vi "ReadFirmwareVersion.vi"(8 "error in (no error)":errorcluster, 11 "GrovePi in":refnum<class "GrovePi.lvclass">) -> (0 "error out":errorcluster, 2 "Firmware Version":string, 3 "GrovePi out":refnum<class "GrovePi.lvclass">)   [LabVIEW 2014, in "GrovePi.lvclass"]
doc: "Returns the Firmware Version of the GrovePi"
uses:
  GrovePi.lvclass
  Command.ctl
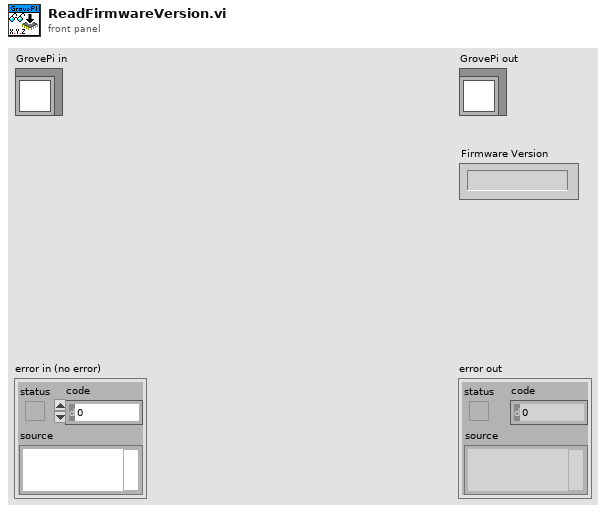
[diagram p1: front panel]
types:
  T1 = typedef "GrovePi.lvclass/Command.ctl" = u8
  T2 = cluster{"Message[0]":u8, "Message[1]":u8, "Message[2]":u8, "Message[3]":u8}
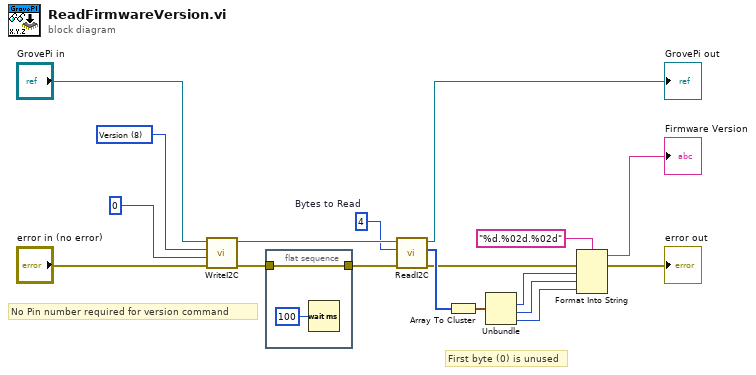
[diagram p0: block diagram]
diagram:
  w11 = u8 4  # Bytes to Read
  w16 = T1 8 items=["Digital Read"=1, "Digital Write"=2, "Analog Read"=3, "Analog Write"=4, "Pin Mode"=5, "Ultrasonic Read"=7, "Version"=8, "Dust Sensor Read"=10, "Encoder Read"=11, "Flow Read"=12, "Flow Disabled"=13, "Dust Sensor Enable"=14, "Dust Sensor Disable"=15, "Encoder Enable"=16, "Encoder Disable"=17, "Flow Enable"=18, "Accelerometer Read"=20, "RTC Read"=30, "DHT Read"=40] ("Command")
  # "First byte (0) is unused"
  # "No Pin number required for version command"
  n1 = call "WriteI2C.vi"("error in (no error)"="error in (no error)", "Pin"=u8 0, "Command"=w16, "GrovePi in"="GrovePi in") -> ("error out"=w14:errorcluster, "GrovePi out"=w12:refnum<class "GrovePi.lvclass">)  [unwired: 5 in, 1 out]
  n2 = flat-sequence {
    tunnel: w14 -> [w19]
    tunnel: [w19] -> w13
    frame #0 {
      n3 = Wait (ms)(milliseconds to wait=u32 100) -> ()  [unwired: 1 out]
    }
  }
  n4 = call "ReadI2C.vi"("error in (no error)"=w13, "Bytes to Read"=w11, "GrovePi in"=w12) -> ("error out"=w7:errorcluster, "Message"=w9:u8[], "GrovePi out"=→"GrovePi out":refnum<class "GrovePi.lvclass">)  [unwired: 6 in]
  n5 = Array To Cluster(array=w9) -> (cluster=w8:T2)
  n6 = Unbundle(w8) -> ("Message[1]"=w3:u8, "Message[2]"=w2:u8, "Message[3]"=w1:u8)  [unwired: 1 out]
  n7 = Format Into String(format string="%d.%02d.%02d", error in=w7, w3, w2, w1) -> (resulting string=→"Firmware Version":string, error out=→"error out":errorcluster)  [unwired: 1 in]
